vi "Write to NT.vi"   [LabVIEW 2020]
uses:
  <vilib>/Rock Robotics/Network Tables/NT Write Boolean.vi
  Globals/Turret_Globals.vi
  Globals/Flywheel_Globals.vi
  Globals/Calibration_And_Constant_Globals.vi
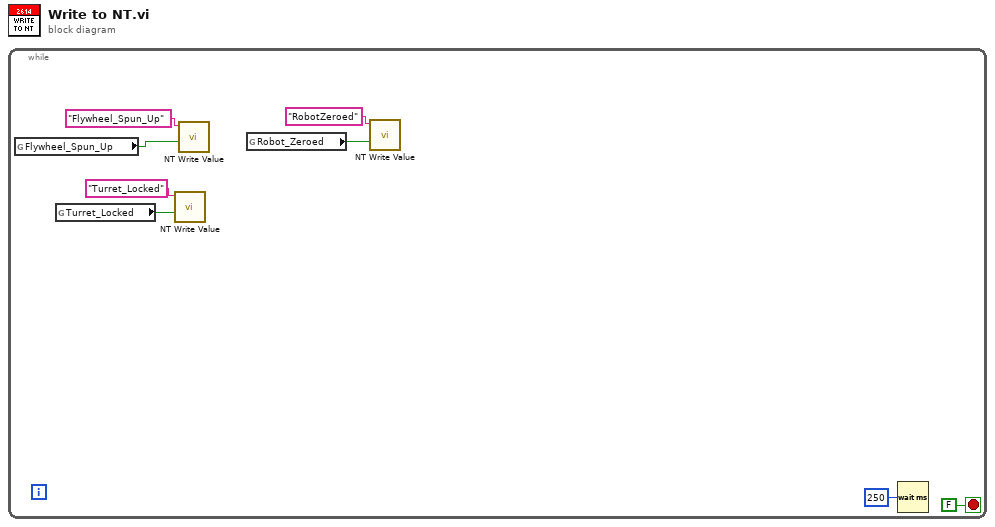
[diagram p0: block diagram]
diagram:
  n1 = while {
    stop <- FALSE stop-if-true
    n2 = global read "Flywheel_Globals.vi" "Flywheel_Spun_Up"() -> (w6:bool)
    n3 = global read "Turret_Globals.vi" "Turret_Locked"() -> (w8:bool)
    n4 = call-poly <vilib>:"NT Write Value.vi"("Boolean"=w8, "Name"="Turret_Locked") -> ()  [unwired: 9 in, 1 out]
    n5 = call-poly <vilib>:"NT Write Value.vi"("Boolean"=w6, "Name"="Flywheel_Spun_Up") -> ()  [unwired: 9 in, 1 out]
    n6 = global read "Calibration_And_Constant_Globals.vi" "Robot_Zeroed"() -> (w3:bool)
    n7 = call-poly <vilib>:"NT Write Value.vi"("Boolean"=w3, "Name"="RobotZeroed") -> ()  [unwired: 9 in, 1 out]
    n8 = Wait (ms)(milliseconds to wait=u32 250) -> ()  [unwired: 1 out]
  }
